vi "control_elo.vi"(8 "error in (no error)":errorcluster, 9 "Numeric":dbl, 10 "all rows":dbl[](array[numeric]), 11 "VISA Refnum in":refnum<visa-resource-name>) -> (0 "error out":errorcluster, 3 "VISA Refnum out":refnum<visa-resource-name>)   [LabVIEW 2019]
uses:
  <instrlib>/Kikusui PLZ 4W Series/Kikusui PLZ 4W Series.lvlib
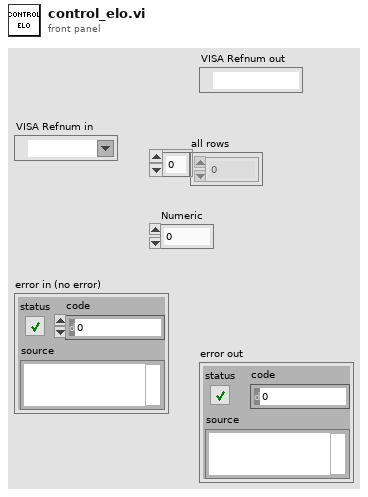
[diagram p1: front panel]
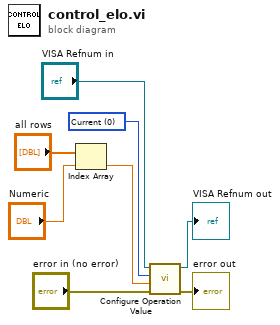
[diagram p0: block diagram]
diagram:
  w4 = u16 0 items=["Current", "Voltage", "Power", "Conductance"] ("Value Type (0:Current)")
  n1 = Index Array(array="all rows", index="Numeric") -> (element=w1:dbl)
  n2 = call <instrlib>:"Configure Operation Value.vi"("error in (no error)"="error in (no error)", "Values (0)"=w1, "Value Type (0:Current)"=w4, "VISA resource name"="VISA Refnum in") -> ("error out"=→"error out":errorcluster, "VISA resource name out"=→"VISA Refnum out":refnum<visa-resource-name>)  [unwired: 6 in]
